vi "Counter Input.vi"(7 "Read Value? (F)":bool, 8 "error in (no error)":errorcluster, 9 "Counter Input (INPUT 1)":T1=enum."INPUT 1", 10 "Counter (A)":T2, 11 "VISA resource name":refnum<visa-resource-name>) -> (0 "error out":errorcluster, 1 "Counter Input":T1=enum."INPUT 1", 3 "VISA resource name out":refnum<visa-resource-name>)   [LabVIEW 2013, in "SRS SR400.lvlib"]
doc: "<B>CI i { ,j }</B>\n\nThe CI command sets and reads the counter inputs. i = 0, 1, or 2 selecting counter A,B, or T and is required. If j is included, then the input to counter i is changed to source j. If j is absent, the input to counter i is \nreturned.\n\n<B>j Input</B>\n0 10 MHz\n1 INPUT 1\n2 INPUT 2\n3 TRIG\n\n<B>Counter Allowed Inputs</B>\nA 10 MHz, INPUT1\nB INPUT 1, INPUT 2\nT 10 MHz, INPUT 2, TRIG\n\nChanging a counter input while counting may result in bad count data."
uses:
  <instrlib>/SRS SR400/SRS SR400.lvlib
  <instrlib>/SRS SR400/Public/Typedefs/Counter.ctl
  <instrlib>/SRS SR400/Public/Typedefs/Counter Input.ctl
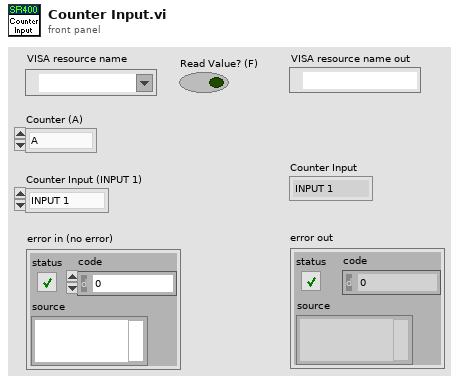
[diagram p1: front panel]
types:
  T1 = typedef "SRS SR400.lvlib/Counter Input.ctl" = enum16{"10 MHz", "INPUT 1", "INPUT 2", "TRIG"}
  T2 = typedef "SRS SR400.lvlib/Counter.ctl" = enum16{"A", "B", "T"}
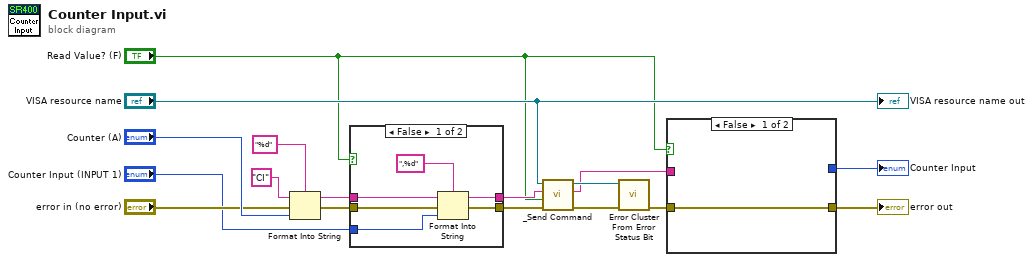
[diagram p0: block diagram]
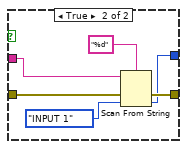
[diagram p2: hidden frame]
diagram:
  n1 = Format Into String(format string="%d", initial string="CI" ("command"), error in="error in (no error)", "Counter (A)") -> (resulting string=w14:string, error out=w13:errorcluster)
  n2 = case shown="False" "Read Value? (F)" {
    tunnel: w14 -> [w18 w24]
    tunnel: w13 -> [w22 w25]
    tunnel: [w21 w24] -> w11
    tunnel: [w20 w25] -> w10
    tunnel: "Counter Input (INPUT 1)" -> [w19 _]
    frame False {
      n3 = Format Into String(format string=",%d", initial string=w18, error in=w22, w19) -> (resulting string=w21:string, error out=w20:errorcluster)
    }
    frame True {
    }
  }
  n4 = call <instrlib>:"_Send Command.vi"("error in (no error)"=w10, "Read Value? (F)"="Read Value? (F)", "Command"=w11, "VISA resource name"="VISA resource name") -> ("error out"=w8:errorcluster, "Response"=w3:string, "VISA resource name out"=w7:refnum<visa-resource-name>)  [unwired: 5 out]
  n5 = call <instrlib>:"Error Cluster From Error Status Bit.vi"("error in (no error)"=w8, "VISA resource name"=w7) -> ("error out"=w5:errorcluster)  [unwired: 8 in, 1 out]
  n6 = case shown="False" "Read Value? (F)" {
    tunnel: [w26 w31] -> w4
    tunnel: w5 -> [w26 w32]
    tunnel: w3 -> [_ w29]
    tunnel: [_ w28] -> w1
    frame False {
    }
    frame True {
      n7 = Scan From String(format string="%d", input string=w29, error in=w32, default 1=Counter_Input."INPUT 1" ("Counter Input (10MHz)")) -> (error out=w31:errorcluster, output 1=w28:T1)  [unwired: 1 in, 2 out]
    }
  }
  "error out" <- w4
  "Counter Input" <- w1
  "VISA resource name out" <- "VISA resource name"
